vi "Write Value.vi"(8 "error in (no error)":errorcluster, 9 "Value":variant, 10 "Data Name (Use Value Name)":string, 11 "Current Value Table":T1) -> (0 "error out":errorcluster, 3 "Current Value Table":T1)   [LabVIEW 2015, in "CurrentValueTable.lvlib" / "CurrentValueTable.lvclass"]
uses:
  CurrentValueTable.lvclass
  CurrentValueTable Reference.ctl
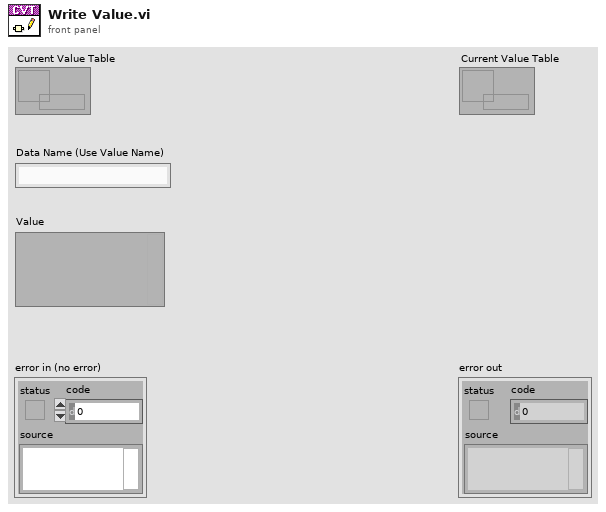
[diagram p1: front panel]
types:
  T1 = typedef "CurrentValueTable.lvlib/CurrentValueTable.lvclass/CurrentValueTable Reference.ctl" = refnum<data-value>
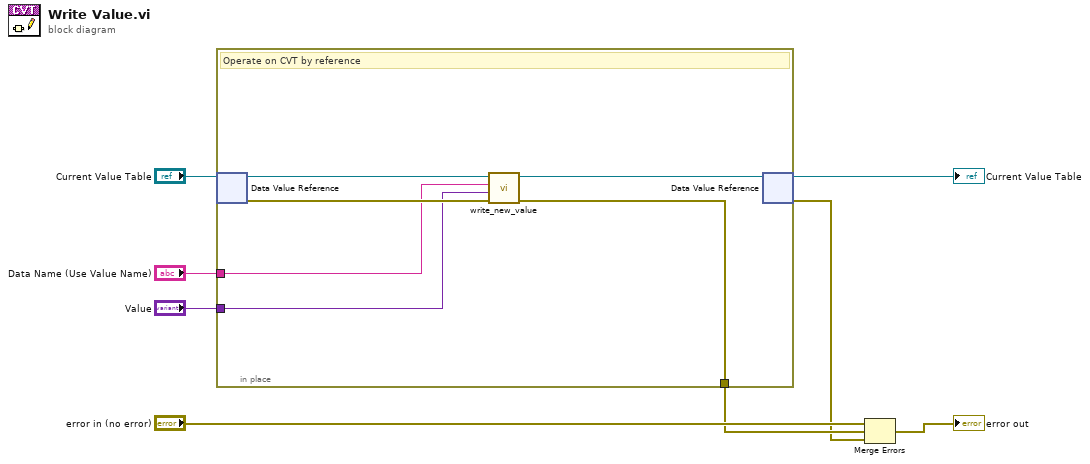
[diagram p0: block diagram]
diagram:
  n1 = in-place {
    in-place-border: [w11] -> w4
    in-place-border: "Value" -> [w9]
    in-place-border: "Data Name (Use Value Name)" -> [w10]
    # "Operate on CVT by reference"
    n2 = in-place-dvr #1("Current Value Table") -> (w14:refnum<class "CurrentValueTable.lvclass">, w12:errorcluster)
    n3 = call "write_new_value.vi"("error in (no error)"=w12, "Value"=w9, "Data Name (Use Value Name)"=w10, "CurrentValueTable in"=w14) -> ("error out"=w11:errorcluster, "CurrentValueTable out"=w13:refnum<class "CurrentValueTable.lvclass">)  [unwired: 6 in]
    n4 = in-place-dvr #1(w13) -> (→"Current Value Table":T1, w3:errorcluster)
  }
  n5 = Merge Errors("error in (no error)", w4, w3) -> (→"error out":errorcluster)
